vi "XYZtoLab.vi"(1 "XrYrZr":dbl[](array[numeric]), 2 "XYZ":dbl[](array[numeric])) -> (0 "L*a*b*":dbl[](array[numeric]))   [LabVIEW 2014]
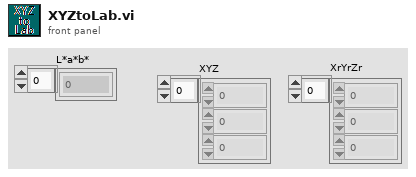
[diagram p1: front panel]
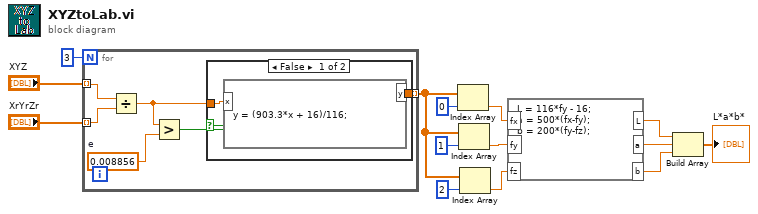
[diagram p0: block diagram]
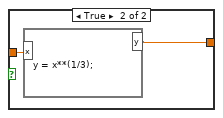
[diagram p2: hidden frame]
diagram:
  n1 = for {
    N: 3 -> [_]
    tunnel: "XYZ" -> [w20] mode=indexing
    tunnel: "XrYrZr" -> [w19] mode=indexing
    tunnel: [w15] -> w10 mode=indexing
    w18 = 0.008856  # e
    n2 = Divide(x=w20, y=w19) -> (x/y=w16:dbl)
    n3 = Greater?(x=w16, y=w18) -> (0:w17:bool)
    n4 = case shown="False" w17 {
      tunnel: w16 -> [w22 w24]
      tunnel: [w21 w23] -> w15
      frame False {
        n5 = formula code="y = (903.3*x + 16)/116;"("x"=w22) -> ("y"=w21:dbl)
      }
      frame True {
        n6 = formula code="y = x**(1/3);"("x"=w24) -> ("y"=w23:dbl)
      }
    }
  }
  n7 = Index Array(array=w10, index=0) -> (element=w7:dbl)
  n8 = Index Array(array=w10, index=1) -> (element=w6:dbl)
  n9 = Index Array(array=w10, index=2) -> (element=w5:dbl)
  n10 = formula code="L = 116*fy - 16;\na = 500*(fx-fy);\nb = 200*(fy-fz);"("fx"=w7, "fy"=w6, "fz"=w5) -> ("L"=w4:dbl, "a"=w3:dbl, "b"=w2:dbl)
  n11 = Build Array(w4, w3, w2) -> (→"L*a*b*":dbl[])
